vi "Read NPSV RT FIFO-Write to Q2.vi"(8 "error in (no error)":errorcluster, 10 "milliseconds to wait":u32, 11 "Q2 IN":T1) -> (0 "error IO":errorcluster, 2 "Q2 timed out?":bool, 3 "Q2 OUT":T1)   [LabVIEW 2016]
uses:
  Q2 Control.ctl
  Queue2 Cluster Control.ctl
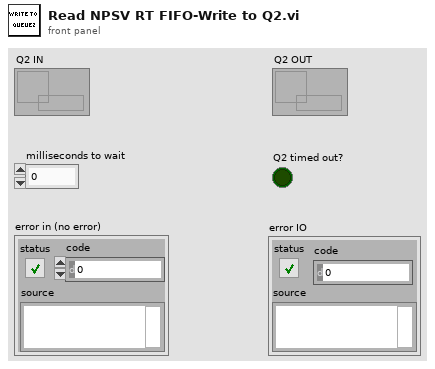
[diagram p1: front panel]
types:
  T1 = typedef "Q2 Control.ctl" = refnum<queue>
  T2 = typedef "Queue2 Cluster Control.ctl" = cluster{"Time till T_u":u32[], "Time till T_u Timestamp":timestamp, "Final Step":u16[], "Final Step Timestamp":timestamp}
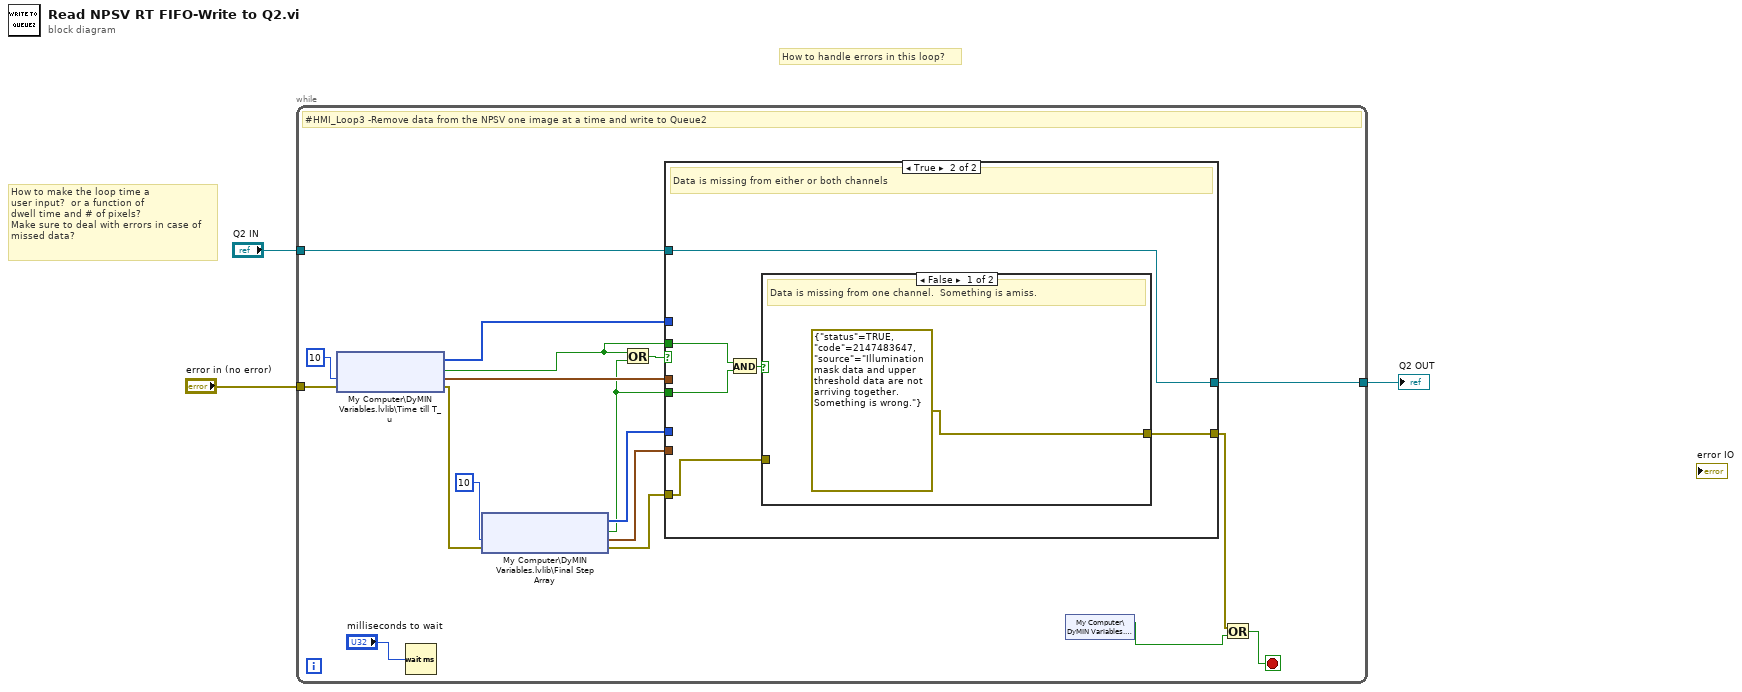
[diagram p0: block diagram]
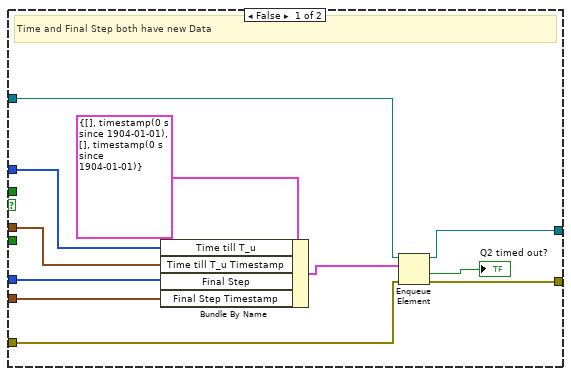
[diagram p2: hidden frame]
diagram:
  # "How to handle errors in this loop?"
  # "How to make the loop time a\nuser input?  or a function of\ndwell time and # of pixels?\nMake sure to deal with errors in case of\nmissed data?"
  n1 = while {
    tunnel: "error in (no error)" -> [w21]
    tunnel: "Q2 IN" -> [w12]
    tunnel: [w4] -> w1
    stop <- w7 stop-if-true
    # "#HMI_Loop3 -Remove data from the NPSV one image at a time and write to Queue2"
    n2 = shared-variable "My Computer\\DyMIN Variables.lvlib\\Time till T_u"(error in=w21, 10 ("ms timeout (0)")) -> (w17:u32[], error out=w20:errorcluster, w16:timestamp, w6:bool)
    n3 = Wait (ms)(milliseconds to wait="milliseconds to wait") -> ()  [unwired: 1 out]
    n4 = shared-variable "My Computer\\DyMIN Variables.lvlib\\Final Step Array"(error in=w20, 10 ("ms timeout (0)")) -> (w14:u16[], error out=w11:errorcluster, w5:bool, w13:timestamp)
    n5 = Or(x=w6, y=w5) -> (x .or. y?=w15:bool)
    n6 = case shown="True" w15 {
      tunnel: w17 -> [w32 _]
      tunnel: w16 -> [w30 _]
      tunnel: w14 -> [w29 _]
      tunnel: w13 -> [w28 _]
      tunnel: w12 -> [w26 w33]
      tunnel: w11 -> [w25 w35]
      tunnel: [w24 w34] -> w8
      tunnel: w6 -> [_ w38]
      tunnel: w5 -> [_ w37]
      tunnel: [w22 w33] -> w4
      frame False {
        # "Time and Final Step both have new Data"
        n7 = Bundle By Name(cluster=T2 {"Time till T_u"=[], "Time till T_u Timestamp"=timestamp(0 s since 1904-01-01), "Final Step"=[], "Final Step Timestamp"=timestamp(0 s since 1904-01-01)} ("input cluster"), "Time till T_u"=w32, "Time till T_u Timestamp"=w30, "Final Step"=w29, "Final Step Timestamp"=w28) -> (w27:T2)
        n8 = Enqueue Element(queue=w26, element=w27, error in (no error)=w25) -> (queue out=w22:T1, timed out?=→"Q2 timed out?":bool, error out=w24:errorcluster)  [unwired: 1 in]
      }
      frame True {
        # "Data is missing from either or both channels"
        n9 = And(x=w38, y=w37) -> (x .and. y?=w36:bool)
        n10 = case shown="False" w36 {
          tunnel: w35 -> [_ w40]
          tunnel: [errorcluster {"status"=TRUE, "code"=2147483647, "source"="Illumination mask data and upper threshold data are not arriving together.  Something is wrong."} ("error constant") w40] -> w34
          frame False {
            # "Data is missing from one channel.  Something is amiss."
          }
          frame True {
            # "Data missing from both channels.  All is well."
          }
        }
      }
    }
    n11 = shared-variable "My Computer\\DyMIN Variables.lvlib\\Stop"() -> (w9:bool)  [unwired: 1 in, 1 out]
    n12 = Or(x=w8, y=w9) -> (x .or. y?=w7:bool)
  }
  "Q2 OUT" <- w1
